vi "Read Polling Period, ms.vi"(8 "error in (no error)":errorcluster, 11 "Base Hardware in":refnum<class "Base Hardware.lvclass">) -> (0 "error out":errorcluster, 2 "Polling Period, ms":i64=-1, 3 "Base Hardware out":refnum<class "Base Hardware.lvclass">)   [LabVIEW 2023, in "Abstract Hardware.lvlib" / "Base Hardware.lvclass"]
uses:
  Base Hardware.lvclass
  Base Hardware.lvclass/Base Hardware.ctl
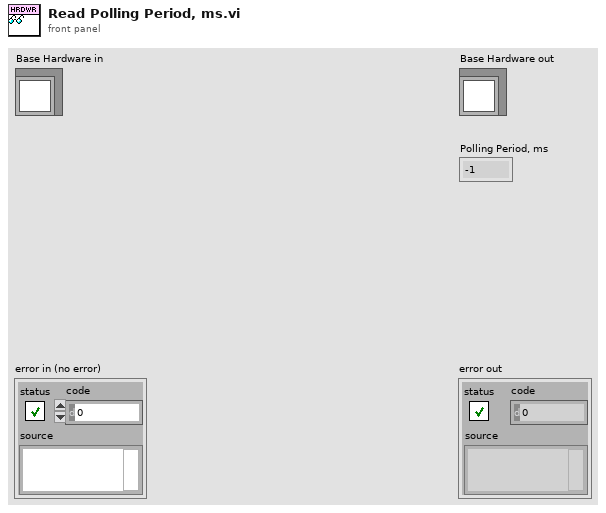
[diagram p1: front panel]
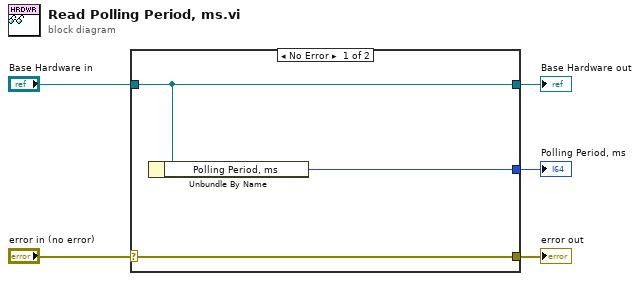
[diagram p0: block diagram]
diagram:
  n1 = case shown="No Error" "error in (no error)" {
    selector: "error in (no error)" -> [w8 w9]
    tunnel: [w8 w9] -> w4
    tunnel: [w7 w10] -> w2
    tunnel: "Base Hardware in" -> [w7 w10]
    tunnel: [w6 _] -> w1
    frame No Error {
      n2 = Unbundle By Name(w7) -> ("Polling Period, ms"=w6:i64)
    }
    frame Error {
    }
  }
  "error out" <- w4
  "Base Hardware out" <- w2
  "Polling Period, ms" <- w1
